vi "ASDA-A2_Jog.vi"(8 "error in":errorcluster, 9 "Jog Type":enum16{"CCW", "CW"}(ring), 10 "Jog(RPM)":u32, 11 "Buffer Data In":T1) -> (0 "error out":errorcluster, 3 "Buffer Data Out":T1)   [LabVIEW 2016]
uses:
  Data Def/ASDA-A2_Buffer Data.ctl
  Data Def/ASDA-A2_Write Register Data.ctl
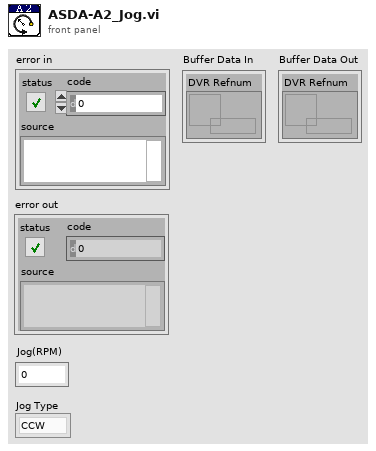
[diagram p1: front panel]
types:
  T1 = typedef "ASDA-A2_Buffer Data.ctl" = cluster{"DVR Refnum":refnum<data-value>}
  T2 = typedef "ASDA-A2_Write Register Data.ctl" = cluster{"Address":u16, "Max Value":u32, "Min Value":u32, "Value":u32, "Type":enum16{"16 Bits", "32 Bits"}, "Page":string, "Description":string}
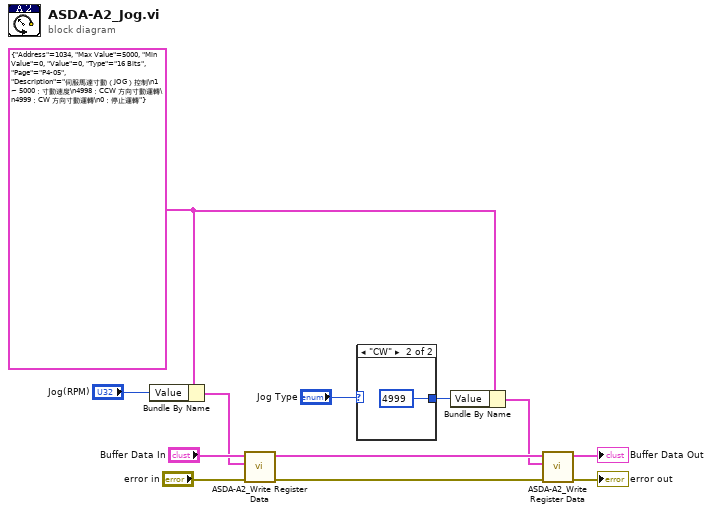
[diagram p0: block diagram]
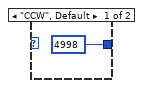
[diagram p2: hidden frame]
diagram:
  w6 = T2 {"Address"=1034, "Max Value"=5000, "Min Value"=0, "Value"=0, "Type"=enum."16 Bits", "Page"="P4-05", "Description"="伺服馬達寸動（JOG）控制\n1 ~ 5000：寸動速度\n4998：CCW 方向寸動運轉\n4999：CW 方向寸動運轉\n0：停止運轉"} ("Write Register Data")
  n1 = Bundle By Name(cluster=w6, "Value"="Jog(RPM)") -> (w9:T2)
  n2 = call "ASDA-A2_Write Register Data.vi"("error in"="error in", "Write Register Data"=w9, "Buffer Data In"="Buffer Data In") -> ("error out"=w8:errorcluster, "Buffer Data Out"=w7:T1)  [unwired: 7 in]
  n3 = case shown="\"CW\"" "Jog Type" {
    tunnel: [u32 4998 u32 4999] -> w3
    frame "CCW", Default {
    }
    frame "CW" {
    }
  }
  n4 = Bundle By Name(cluster=w6, "Value"=w3) -> (w5:T2)
  n5 = call "ASDA-A2_Write Register Data.vi"("error in"=w8, "Write Register Data"=w5, "Buffer Data In"=w7) -> ("error out"=→"error out":errorcluster, "Buffer Data Out"=→"Buffer Data Out":T1)  [unwired: 7 in]
